vi "NI OCR-Event Loop.vi"(8 "error in":errorcluster, 11 "Buffer Data In":T1={"VI Refnum"=refnum, "Src Image"=refnum, "Dst Image"=refnum, "Ctl Refnum []"=[], "Ctl Label"=[], "User Event"=refnum, "Event Registration Refnum"=refnum, "Timeout"=0, "IMAQ OCR Session"=refnum, "Objects"=[], "ROI Descriptor"={"Global Rectangle"=[], "Contours"=[]}, "Settings"={"Objects"=0, "Threshold"=128, "Reject Border"=FALSE, "Fill Holes"=FALSE, "Min Object Size"=FALSE, "Min Size"=3, "Max Object Size"=FALSE, "Max Size"=100, "Show Search Area"=FALSE, "Show Center"=TRUE, "Show Bounding Box"=TRUE}} {"Settings"."Objects" items=["Bright Objects", "Dark Objects"]; "Settings"."Threshold" min=1 max=999999999 step=1; "Settings"."Max Size" min=1 max=999999999 step=1; "Settings"."Min Size" min=1 max=999999999 step=1; "ROI Descriptor"."Contours"."Type" items=["No Selection", "Point", "Line", "Rectangle", "Oval", "Polygon", "Freehand Region", "Annulus", "Unused2", "Unused3", "Broken Line", "Freehand Line", "Rotated Rectangle"]; "Objects"."Aspect Ratio" format="%.2f"; "Objects"."Orientation" format="%.2f"; "Objects"."Area" format="%.2f"; "Objects"."Object Center"."Y" format="%.2f"; "Objects"."Object Center"."X" format="%.2f"}) -> (0 "error out":errorcluster, 3 "Buffer Data Out":T1={"VI Refnum"=refnum, "Src Image"=refnum, "Dst Image"=refnum, "Ctl Refnum []"=[], "Ctl Label"=[], "User Event"=refnum, "Event Registration Refnum"=refnum, "Timeout"=0, "IMAQ OCR Session"=refnum, "Objects"=[], "ROI Descriptor"={"Global Rectangle"=[], "Contours"=[]}, "Settings"={"Objects"=0, "Threshold"=128, "Reject Border"=FALSE, "Fill Holes"=FALSE, "Min Object Size"=FALSE, "Min Size"=3, "Max Object Size"=FALSE, "Max Size"=100, "Show Search Area"=FALSE, "Show Center"=TRUE, "Show Bounding Box"=TRUE}} {"Settings"."Objects" items=["Bright Objects", "Dark Objects"]; "Settings"."Threshold" min=1 max=999999999 step=1; "Settings"."Max Size" min=1 max=999999999 step=1; "Settings"."Min Size" min=1 max=999999999 step=1; "ROI Descriptor"."Contours"."Type" items=["No Selection", "Point", "Line", "Rectangle", "Oval", "Polygon", "Freehand Region", "Annulus", "Unused2", "Unused3", "Broken Line", "Freehand Line", "Rotated Rectangle"]; "Objects"."Aspect Ratio" format="%.2f"; "Objects"."Orientation" format="%.2f"; "Objects"."Area" format="%.2f"; "Objects"."Object Center"."Y" format="%.2f"; "Objects"."Object Center"."X" format="%.2f"})   [LabVIEW 2016]
uses:
  Data Def/NI OCR-Buffer Data.ctl
  <vilib>/vision/Image Controls.llb/IMAQ Image.ctl
  Data Def/NI OCR-User Event Data.ctl
  <vilib>/vision/OCR.llb/IMAQ OCR Session.ctl
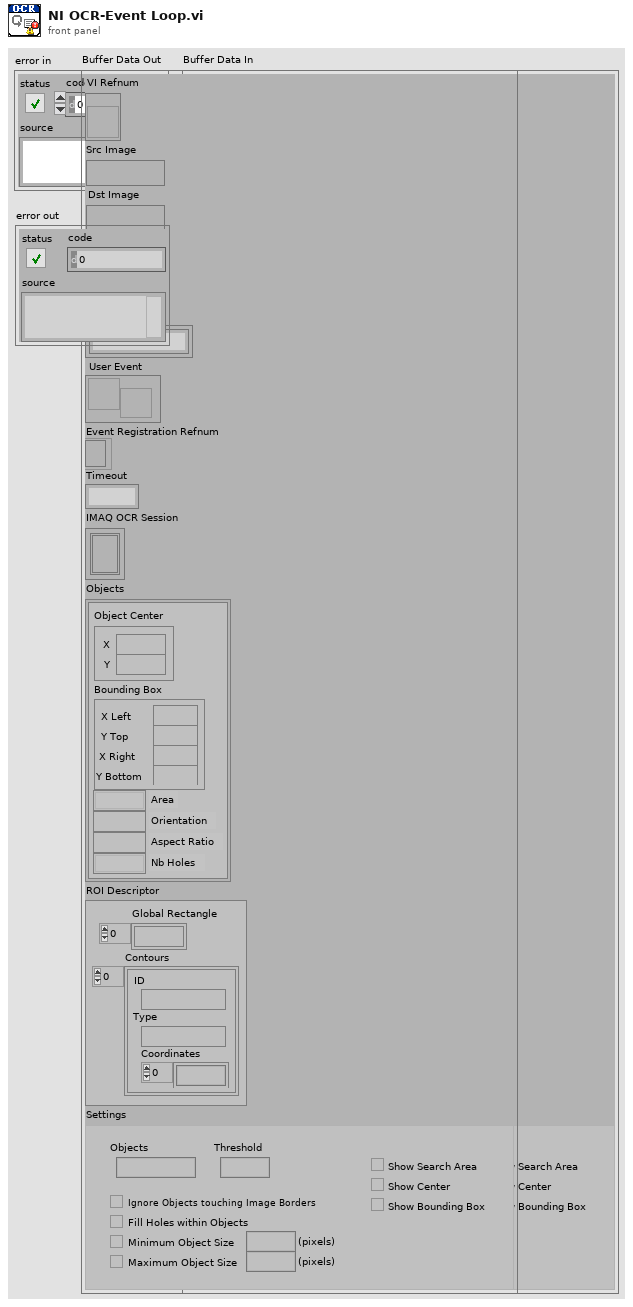
[diagram p1: front panel]
types:
  T1 = typedef "NI OCR-Buffer Data.ctl" = cluster{"VI Refnum":refnum<vi>, "Src Image":T2, "Dst Image":T2, "Ctl Refnum []":refnum<vi>[], "Ctl Label":string[], "User Event":refnum<user-event>, "Event Registration Refnum":refnum<event-registration>, "Timeout":i32, "IMAQ OCR Session":T3, "Objects":cluster{"Object Center":cluster{"X":sgl, "Y":sgl}, "Bounding Box":cluster{"X Left":i32, "Y Top":i32, "X Right":i32, "Y Bottom":i32}, "Area":sgl, "Orientation":sgl, "Aspect Ratio":sgl, "Nb Holes":i32}[], "ROI Descriptor":T4, "Settings":cluster{"Objects":u16, "Threshold":i32, "Reject Border":bool, "Fill Holes":bool, "Min Object Size":bool, "Min Size":i32, "Max Object Size":bool, "Max Size":i32, "Show Search Area":bool, "Show Center":bool, "Show Bounding Box":bool}}
  T2 = typedef "IMAQ Image.ctl" = refnum<image>
  T3 = typedef "IMAQ OCR Session.ctl" = refnum<k1>
  T4 = typedef "ROI Descriptor" = cluster{"Global Rectangle":i32[], "Contours":cluster{"ID":enum32{"External", "Internal"}, "Type":u32, "Coordinates":i32[]}[]}
  T5 = typedef "NI OCR-User Event Data.ctl" = cluster{"Command":string, "Data":variant}
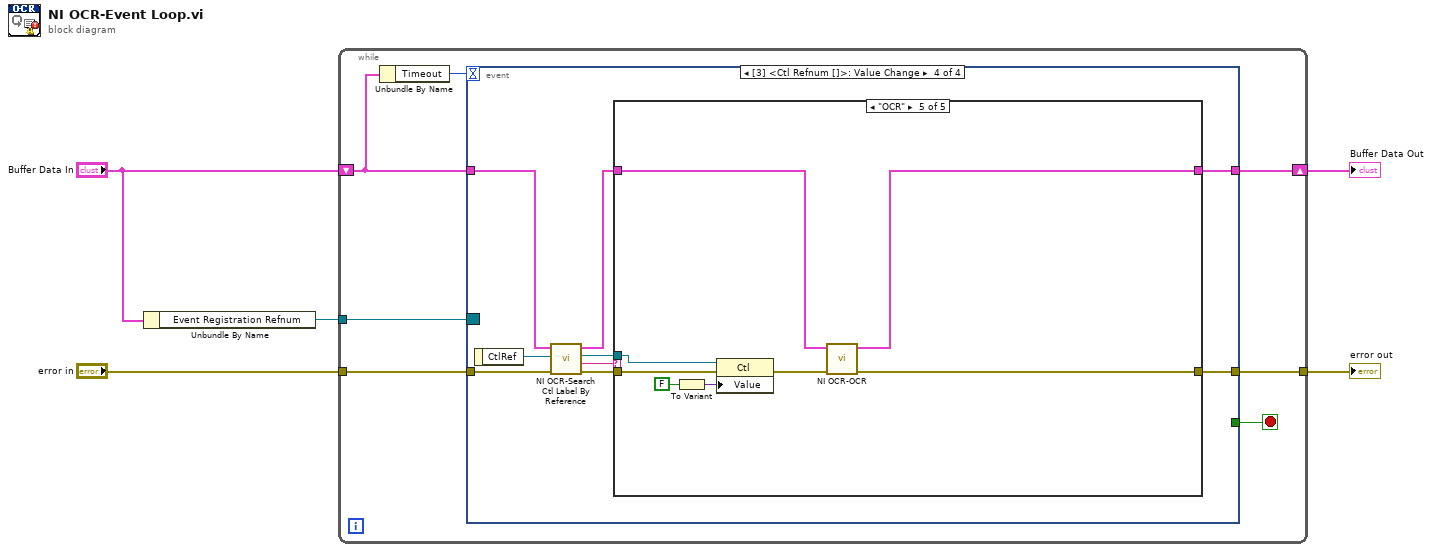
[diagram p0: block diagram]
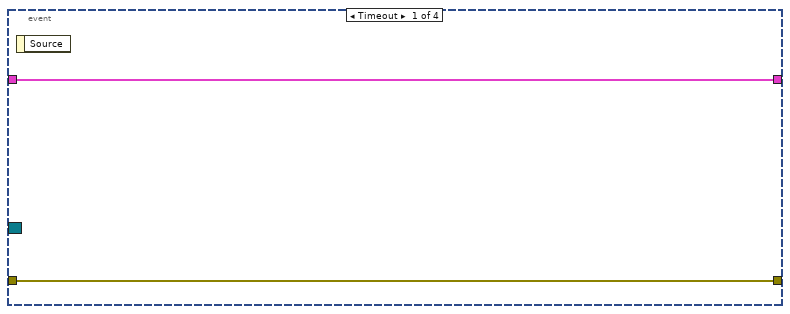
[diagram p2: hidden frame]
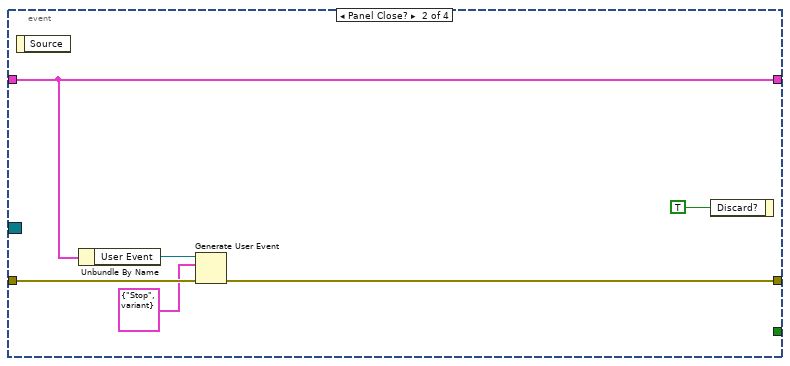
[diagram p3: hidden frame]
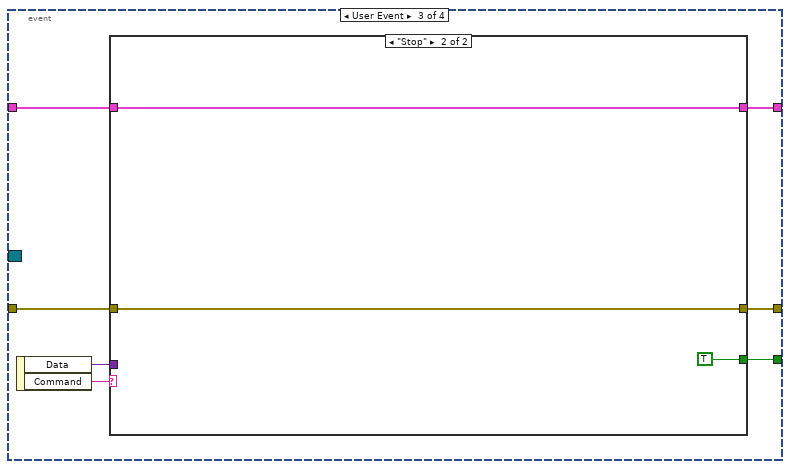
[diagram p4: hidden frame]
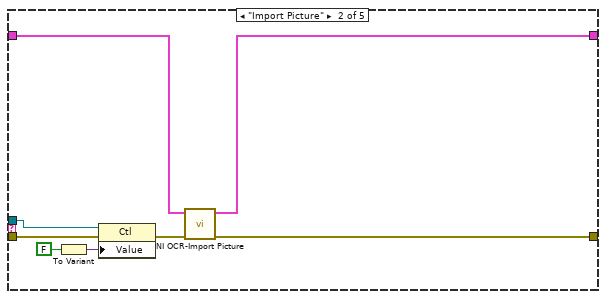
[diagram p7: hidden frame]
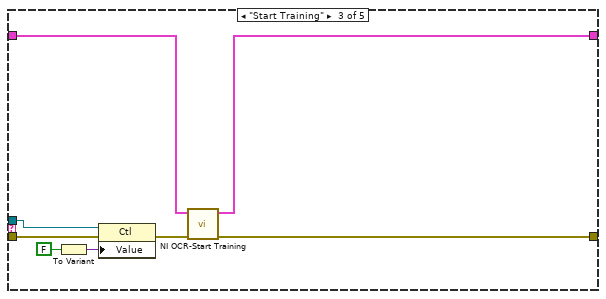
[diagram p8: hidden frame]
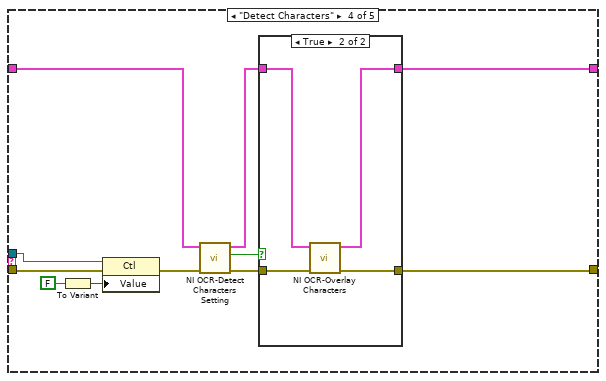
[diagram p9: hidden frame]
diagram:
  n1 = Unbundle By Name("Buffer Data In") -> ("Event Registration Refnum"=w5:refnum<event-registration>)
  n2 = while {
    tunnel: w5 -> [w12]
    shift-right: [w8] -> w2
    shift-left: "Buffer Data In" -> [w11]
    tunnel: "error in" -> [w9]
    tunnel: [w7] -> w1
    stop <- w6 stop-if-true
    n3 = Unbundle By Name(w11) -> ("Timeout"=w10:i32)
    n4 = event shown="[3] <Ctl Refnum []>: Value Change" {
      selector: w12 -> [_ _ _ _]
      dyn-events: _ -> [_ _ _ _]
      timeout: w10 -> [_ _ _ _]
      tunnel: w11 -> [w14 w19 w24 w39]
      tunnel: w9 -> [w13 w18 w25 w41]
      tunnel: [w14 w19 w23 w37] -> w8
      tunnel: [w13 w16 w22 w35] -> w7
      tunnel: [_ _ w21 _] -> w6
      event Timeout {
        n5 = event-data() -> ()  [unwired: 1 in, 1 out]
      }
      event Panel Close? {
        n6 = event-data() -> ()  [unwired: 1 in, 1 out]
        n7 = Unbundle By Name(w19) -> ("User Event"=w17:refnum<user-event>)
        n8 = Generate User Event(user event=w17, event data cluster=T5 {"Command"="Stop", "Data"=variant} ("event data"), error in=w18) -> (error out=w16:errorcluster)  [unwired: 1 in, 1 out]
        n9 = event-data("Discard?"=TRUE) -> ()  [unwired: 1 in, 1 out]
      }
      event User Event {
        n10 = event-data() -> ("Data"=w26:variant, "Command"=w27:string)  [unwired: 1 in]
        n11 = case shown="\"Stop\"" w27 {
          tunnel: w26 -> [_ _]
          tunnel: w25 -> [w28 w31]
          tunnel: w24 -> [w29 w32]
          tunnel: [w29 w32] -> w23
          tunnel: [w28 w31] -> w22
          tunnel: [_ TRUE] -> w21
          frame Default {
          }
          frame "Stop" {
          }
        }
      }
      event Value Change {
        n12 = event-data() -> ("CtlRef"=w40:refnum<vi>)  [unwired: 1 in]
        n13 = call "NI OCR-Search Ctl Label By Reference.vi"("error in"=w41, "Ctl Refnum In"=w40, "Buffer Data In"=w39) -> ("error out"=w36:errorcluster, "Ctl Label"=w34:string, "Ctl Refnum Out"=w33:refnum<vi>, "Buffer Data Out"=w38:T1)  [unwired: 5 in]
        n14 = case shown="\"OCR\"" w34 {
          tunnel: w38 -> [w42 w46 w54 w65 w84]
          tunnel: [w42 w44 w53 w61 w83] -> w37
          tunnel: w36 -> [w43 w51 w59 w68 w79]
          tunnel: [w43 w45 w52 w60 w82] -> w35
          tunnel: w33 -> [_ w50 w58 w67 w78]
          frame Default {
          }
          frame "Import Picture" {
            n15 = To Variant(anything=FALSE) -> (Variant=w49:variant)
            n16 = property class="Ctl"(reference=w50, error in=w51, "Value"=w49) -> (error out=w47:errorcluster)  [unwired: 1 out]
            n17 = call "NI OCR-Import Picture.vi"("error in"=w47, "Buffer Data In"=w46) -> ("error out"=w45:errorcluster, "Buffer Data Out"=w44:T1)  [unwired: 8 in]
          }
          frame "Start Training" {
            n18 = To Variant(anything=FALSE) -> (Variant=w57:variant)
            n19 = property class="Ctl"(reference=w58, error in=w59, "Value"=w57) -> (error out=w55:errorcluster)  [unwired: 1 out]
            n20 = call "NI OCR-Start Training.vi"("error in"=w55, "Buffer Data In"=w54) -> ("error out"=w52:errorcluster, "Buffer Data Out"=w53:T1)  [unwired: 8 in]
          }
          frame "Detect Characters" {
            n21 = To Variant(anything=FALSE) -> (Variant=w70:variant)
            n22 = property class="Ctl"(reference=w67, error in=w68, "Value"=w70) -> (error out=w66:errorcluster)  [unwired: 1 out]
            n23 = call "NI OCR-Detect Characters Setting.vi"("error in"=w66, "Buffer Data In"=w65) -> ("error out"=w64:errorcluster, "OK?"=w63:bool, "Buffer Data Out"=w62:T1)  [unwired: 7 in]
            n24 = case shown="True" w63 {
              tunnel: w64 -> [w71 w76]
              tunnel: w62 -> [w72 w75]
              tunnel: [w72 w73] -> w61
              tunnel: [w71 w74] -> w60
              frame False {
              }
              frame True {
                n25 = call "NI OCR-Overlay Characters.vi"("error in"=w76, "Buffer Data In"=w75) -> ("error out"=w74:errorcluster, "Buffer Data Out"=w73:T1)  [unwired: 8 in]
              }
            }
          }
          frame "OCR" {
            n26 = To Variant(anything=FALSE) -> (Variant=w81:variant)
            n27 = property class="Ctl"(reference=w78, error in=w79, "Value"=w81) -> (error out=w77:errorcluster)  [unwired: 1 out]
            n28 = call "NI OCR-OCR.vi"("error in"=w77, "Buffer Data In"=w84) -> ("error out"=w82:errorcluster, "Buffer Data Out"=w83:T1)  [unwired: 8 in]
          }
        }
      }
    }
  }
  "Buffer Data Out" <- w2
  "error out" <- w1
